vi "Delete Key.vi"(4 "Return deleted names? [F]":bool, 5 "Key name":string, 7 "Section name":string, 8 "error in (no error)":errorcluster, 9 "Use Key Regex? [F]":bool, 10 "Use Section Regex? [F]":bool, 11 "Carya Config in":refnum<class "Carya Config.lvclass">) -> (0 "error out":errorcluster, 1 "Key names":string[](array[string]), 2 "Section names":string[](array[string]), 3 "Carya Config out":refnum<class "Carya Config.lvclass">)   [LabVIEW 2013, in "Carya Config.lvclass"]
doc: "Copyright 2018, Carya Automatisering, Wiebe Walstra."
uses:
  Carya Config.lvclass
  CConfig Object/Delete Query/Delete Query.lvclass
  CConfig Object/Add Results Query/Add Results Query.lvclass
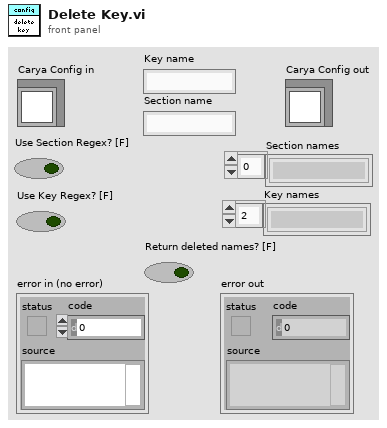
[diagram p1: front panel]
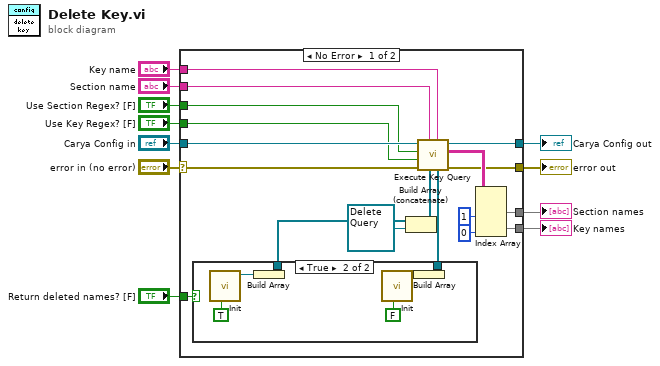
[diagram p0: block diagram]
diagram:
  n1 = case shown="No Error" "error in (no error)" {
    selector: "error in (no error)" -> [w22 w37]
    tunnel: [w21 w37] -> w10
    tunnel: [w20 w36] -> w8
    tunnel: "Carya Config in" -> [w19 w36]
    tunnel: "Section name" -> [w12 _]
    tunnel: "Key name" -> [w13 _]
    tunnel: "Use Section Regex? [F]" -> [w15 _]
    tunnel: "Use Key Regex? [F]" -> [w14 _]
    tunnel: [w29 _] -> w3
    tunnel: [w28 _] -> w2
    tunnel: "Return deleted names? [F]" -> [w18 _]
    frame No Error {
      n2 = case shown="True" w18 {
        tunnel: [_ w31] -> w25
        tunnel: [_ w30] -> w16
        frame False {
        }
        frame True {
          n3 = call "Init.vi"("Concatenate\\Build [T, Concatenate]"=TRUE ("Concatenate\\Build [T, Concatenate]")) -> ("Find First Query out"=w34:refnum<class "Add Results Query.lvclass">)  [unwired: 9 in, 1 out]
          n4 = Build Array(w34) -> (w31:refnum<class "Add Results Query.lvclass">[])
          n5 = call "Init.vi"("Concatenate\\Build [T, Concatenate]"=FALSE ("Concatenate\\Build [T, Concatenate]")) -> ("Find First Query out"=w33:refnum<class "Add Results Query.lvclass">)  [unwired: 9 in, 1 out]
          n6 = Build Array(w33) -> (w30:refnum<class "Add Results Query.lvclass">[])
        }
      }
      n7 = Build Array (concatenate)(w25, refnum<class "Delete Query.lvclass"> refnum ("Delete Query.lvclass")) -> (w17:refnum<class "CConfig Query.lvclass">[])
      n8 = call-dynamic "Execute Key Query.vi"("Section queries"=w16, "Key name"=w13, "Key queries"=w17, "Section name"=w12, "error in (no error)"=w22, "Use Key Regex? [F]"=w14, "Use Section Regex? [F]"=w15, "Carya Config in"=w19) -> ("error out"=w21:errorcluster, "Results"=w26:string[][], "Carya Config out"=w20:refnum<class "Carya Config.lvclass">)  [unwired: 1 in]
      n9 = Index Array(array=w26, index (col) #1=1 ("disabled index (col)"), index (col) #2=0 ("index (col)")) -> (element #1=w29:string[], element #2=w28:string[])  [unwired: 2 in]
    }
    frame Error {
    }
  }
  "error out" <- w10
  "Carya Config out" <- w8
  "Key names" <- w2
  "Section names" <- w3
